vi "Delete empty element from array 复制至S4PVI.vi"(11 "input":string[](array[string])) -> (3 "output":string[](array[string]))   [LabVIEW 2011]
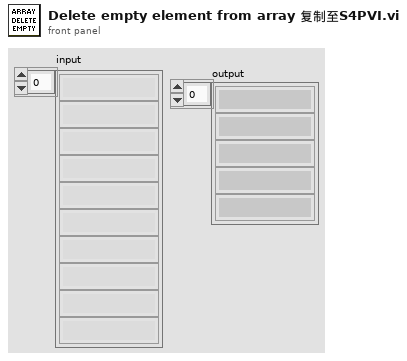
[diagram p1: front panel]
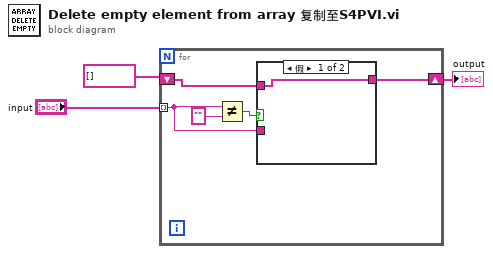
[diagram p0: block diagram]
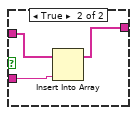
[diagram p2: hidden frame]
diagram:
  n1 = for {
    shift-right: [w4] -> w3
    shift-left: string[] [] ("input") -> [w6]
    tunnel: "input" -> [w5] mode=indexing
    n2 = Not Equal?(x=w5, y="") -> (x != y?=w7:bool)
    n3 = case shown="假" w7 {
      tunnel: w6 -> [w9 w12]
      tunnel: w5 -> [_ w11]
      tunnel: [w9 w10] -> w4
      frame False {
      }
      frame True {
        n4 = Insert Into Array(array=w12, new element=w11) -> (w10:string[])  [unwired: 1 in]
      }
    }
  }
  "output" <- w3
